vi "save configuration.vi"(4 "error in":errorcluster) -> (0 "error":errorcluster, 3 "sensor file path":path)   [LabVIEW 2015]
uses:
  file action.ctl
  DAQ configuration/Sensor buffer command.ctl
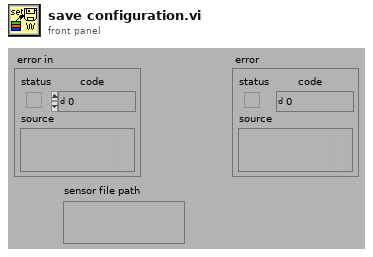
[diagram p1: front panel]
types:
  T1 = typedef "Sensor buffer command.ctl" = enum16{"read average", "read recent", "read all", "write", "set buffer size", "Read channel config", "Write channel config", "clear"}
  T2 = typedef "file action.ctl" = enum16{"Save", "Open"}
  T3 = typedef "Channel config.ctl" = cluster{"Channel Indices":T4[], "AI Max voltage":dbl[], "Calibration matrix":T5}
  T4 = typedef "channel identifier.ctl" = u16
  T5 = typedef "calib array.ctl" = T6[]
  T6 = typedef "conversion.ctl" = cluster{"conversion matrix":sgl[][], "units":string, "name":string, "scale type":T7, "offset (volts)":dbl, "second channel":i8, "correspondence table":T8, "offset (physical units)":dbl, "pH scale":T9, "D.O.":T10, "Photometer data":T11}
  T7 = typedef "scale type.ctl" = enum16{"Volts", "Polynomial", "Correspondence Table", "pH", "Dissolved Oxygen", "Quadratic", "Photometer"}
  T8 = typedef "correspondence table.ctl" = cluster{"physical units":dbl, "volts":dbl}[]
  T9 = typedef "pH scale.ctl" = cluster{"Buffers":cluster{"Buffer":dbl, "Calibrated":bool, "V/T":dbl}[], "Temperature":dbl}
  T10 = typedef "DO scale.ctl" = cluster{"Temperature":dbl, "K":dbl, "barometric pressure":dbl}
  T11 = typedef "Photometer calibration data.ctl" = cluster{"Dark Voltage":dbl, "Blank Voltage":dbl, "Standards":cluster{"Concentration":dbl, "Voltage":dbl}[]}
  T12 = cluster{"Channel Indices":T4[], "Calibration matrix":T5}
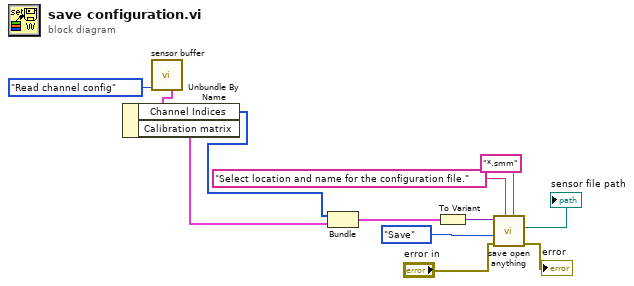
[diagram p0: block diagram]
diagram:
  n1 = call "sensor buffer.vi"("command"=Sensor_buffer_command."Read channel config") -> ("Channel Config out"=w3:T3)  [unwired: 6 in, 4 out]
  n2 = Unbundle By Name(w3) -> ("Channel Indices"=w2:T4[], "Calibration matrix"=w1:T5)
  n3 = Bundle("Channel Indices"=w2, "Calibration matrix"=w1) -> (w12:T12)  [unwired: 1 in]
  n4 = To Variant(anything=w12) -> (Variant=w11:variant)
  n5 = call "save open anything.vi"("Variant"=w11, "Action"=file_action."Save", "error in (not an error)"="error in", "prompt"="Select location and name for the configuration file.", "pattern"="*.smm") -> ("new file path"=→"sensor file path":path, "error out"=→"error":errorcluster)  [unwired: 2 in, 2 out]
